vi "Check PCC for Unintentional Resynchronization.vi"(8 "error in":errorcluster, 11 "Off-Grid in":refnum<class "Off-Grid.lvclass">) -> (0 "error out":errorcluster, 3 "Off-Grid out":refnum<class "Off-Grid.lvclass">)   [LabVIEW 2018, in "Off-Grid Actor.lvlib" / "Off-Grid.lvclass"]
uses:
  Off-Grid.lvclass
  C:/Users/Administrator/Desktop/2018LabVIEW EMS/EMS Generic Actor/EMS Generic/EMS Generic.lvclass
  C:/Users/Administrator/Desktop/2018LabVIEW EMS/Optimization/Generic Optimization Actor/Generic Optimization/Generic Optimization.lvclass
  <vilib>/ORNL/CSEISMIC DDS/CSEISMIC DDS Base/Data Types/Controls/DeviceID.ctl
  <vilib>/ORNL/CSEISMIC DDS/CSEISMIC DDS Base/CSEISMIC DDS.lvclass
  Generic Optimization Actor/Generic Optimization/Generic Optimization.lvclass
  EMS Generic Actor/EMS Generic/EMS Generic.lvclass
  Device Communication and Control Abstract Actor/Device Communication and Control Abstract/Device Communication and Control Abstract.lvclass
  C:/Users/Administrator/Desktop/2018LabVIEW EMS/Device Communication and Control Abstract Actor/Device Communication and Control Abstract/Device Communication and Control Abstract.lvclass
  <vilib>/ORNL/CSEISMIC DDS/CSEISMIC DDS Base/Data Types/Controls/Generation Mode.ctl
  <vilib>/ORNL/CSEISMIC DDS/CSEISMIC DDS Base/Data Types/DER_setGenerationMode.ctl
  Utilities/Status Messaging.llb/Status Messaging.lvlib
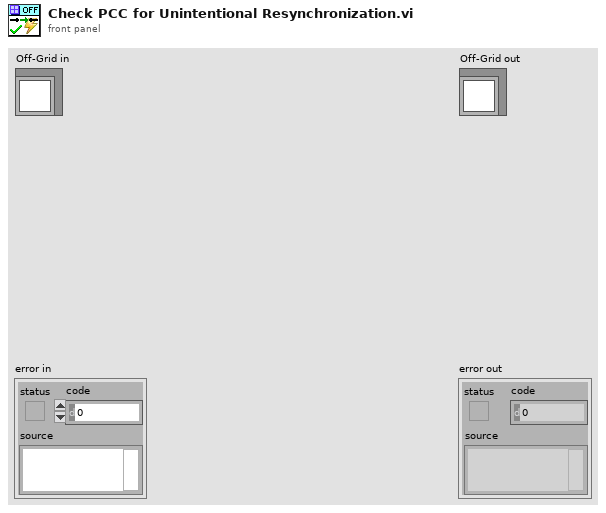
[diagram p1: front panel]
types:
  T1 = typedef "CSEISMIC DDS.lvlib/CSEISMIC DDS.lvclass/DER_setGenerationMode.ctl" = cluster{"DeviceID":T2, "Mode":T3}
  T2 = typedef "CSEISMIC DDS.lvlib/CSEISMIC DDS.lvclass/DeviceID.ctl" = string
  T3 = typedef "CSEISMIC DDS.lvlib/CSEISMIC DDS.lvclass/Generation Mode.ctl" = enum32{"Invalid", "PQ", "Droop", "PV", "PF", "VF"}
  T4 = typedef "CSEISMIC DDS.lvlib/CSEISMIC DDS.lvclass/IED_Status.ctl" = cluster{"DeviceID":T2, "Timestamp":T5, "MicrogridID":u8, "Active":bool, "Inactive":bool, "Error":i32, "Fault":bool, "ErrorString":string}
  T5 = typedef "CSEISMIC DDS.lvlib/CSEISMIC DDS.lvclass/Timestamp.ctl" = cluster{"Seconds":u64, "Remainder":u64}
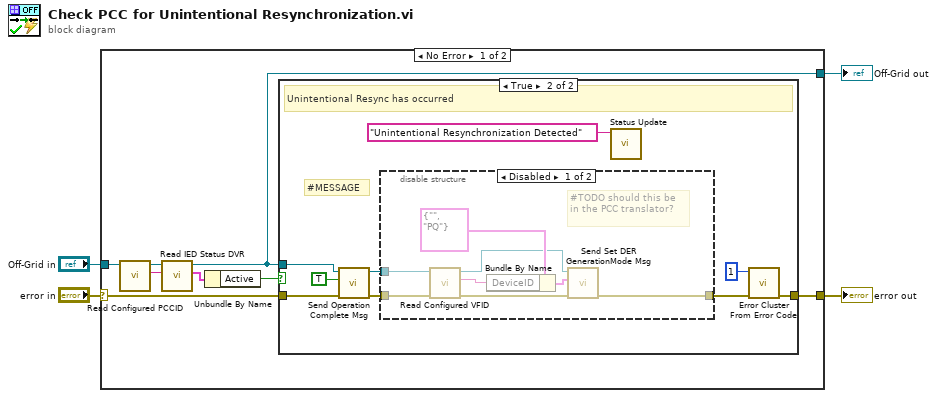
[diagram p0: block diagram]
diagram:
  n1 = case shown="No Error" "error in" {
    selector: "error in" -> [w12 w33]
    tunnel: [w11 w33] -> w3
    tunnel: [w5 w32] -> w1
    tunnel: "Off-Grid in" -> [w9 w32]
    frame No Error {
      n2 = call "Read Configured PCCID.vi"("EMS Generic in"=w9) -> ("PCCID"=w7:T2, "EMS Generic out"=w8:refnum<class "Off-Grid.lvclass">)  [unwired: 8 in, 1 out]
      n3 = call "Read IED Status DVR.vi"("DeviceID"=w7, "EMS Generic in"=w8) -> ("IED_Status"=w6:T4, "EMS Generic out"=w5:refnum<class "Off-Grid.lvclass">)  [unwired: 6 in, 2 out]
      n4 = Unbundle By Name(w6) -> ("Active"=w10:bool)
      n5 = case shown="True" w10 {
        tunnel: w12 -> [w13 w20]
        tunnel: [w13 w22] -> w11
        tunnel: w5 -> [_ w18]
        frame False {
          # "Still offgrid.  Continue as normal."
        }
        frame True {
          # "#MESSAGE"
          # "Unintentional Resync has occurred"
          n6 = call "Send Operation Complete Msg.vi"("error in"=w20, "Operation Complete"=TRUE, "Generic Optimization in"=w18) -> ("error out"=w17:errorcluster, "Generic Optimization out"=w16:refnum<class "Off-Grid.lvclass">)  [unwired: 7 in]
          n7 = disable-structure shown="Disabled" {
            disable-tunnel: w17 -> [w28 w31]
            disable-tunnel: w16 -> [w27 _]
            disable-tunnel: [w23 w31] -> w15
            frame Disabled {
              # "#TODO should this be in the PCC translator?"
              n8 = call "Read Configured VFID.vi"("error in"=w28, "EMS Generic in"=w27) -> ("error out"=w24:errorcluster, "VFID"=w29:T2, "EMS Generic out"=w25:refnum<class "Off-Grid.lvclass">)  [unwired: 7 in]
              n9 = Bundle By Name(cluster=T1 {"DeviceID"="", "Mode"=enum."PQ"} ("DER_setGenerationMode"), "DeviceID"=w29) -> (w26:T1)
              n10 = call "Send Set DER GenerationMode Msg.vi"("error in"=w24, "DER_setGenerationMode"=w26, "SCADA Sub Abstract in"=w25) -> ("error out"=w23:errorcluster)  [unwired: 7 in, 1 out]
            }
            frame Enabled {
            }
          }
          n11 = call "Status Update.vi"("Status Update"="Unintentional Resynchronization Detected") -> ()  [unwired: 9 in, 2 out]
          n12 = call <vilib>:"Error Cluster From Error Code.vi"("error in (no error)"=w15, "error code (0)"=1) -> ("error out"=w22:errorcluster)  [unwired: 7 in]
        }
      }
    }
    frame Error {
    }
  }
  "error out" <- w3
  "Off-Grid out" <- w1
